vi "读取参数.vi"(0 "Slave ID":u8=10, 1 "starting address":u16, 2 "quantity":u16, 3 "Error in":errorcluster caption="Error in (no error)") -> (7 "values":u16[](array[numeric]), 10 "error out":errorcluster)   [LabVIEW 2016, in "质控单元.lvlib"]
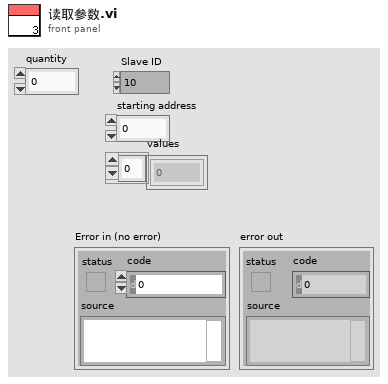
[diagram p1: front panel]
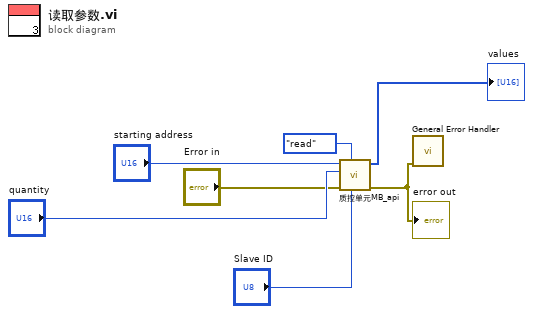
[diagram p0: block diagram]
diagram:
  n1 = call "质控单元MB_api.vi"("Slave ID"="Slave ID", "STEP"=enum16{"open", "read", "write", "close"}."read", "Error in"="Error in", "quantity"="quantity", "starting address"="starting address") -> ("error out"=w1:errorcluster, "Registers"=→"values":u16[])  [unwired: 3 in, 2 out]
  "error out" <- w1
  n2 = call <vilib>:"General Error Handler.vi"("error in (no error)"=w1) -> ()  [unwired: 10 in, 5 out]
